vi "ReadVersion.vi"() -> ()   [LabVIEW 2015]
uses:
  <instrlib>/Ion Motion Roboclaw/Ion Motion Roboclaw.lvlib
panel:
  in  "Address":u8
  out "read buffer":string
  out "valid":bool
  in  "baud rate (38400)":u32
  in  "error in (no error)":errorcluster
  out "error out":errorcluster
  in  "COMPort":refnum<visa-resource-name>
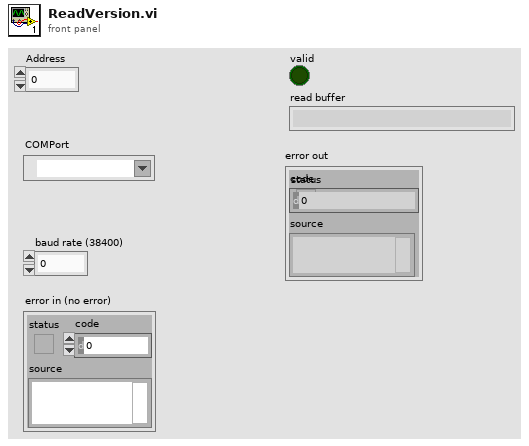
[diagram p1: front panel]
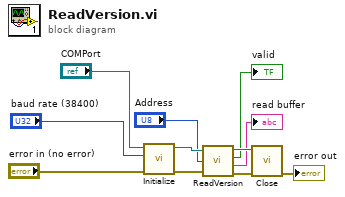
[diagram p0: block diagram]
diagram:
  n1 = call <instrlib>:"Initialize.vi"("error in (no error)"="error in (no error)", "baud rate (38400)"="baud rate (38400)", "COM port"="COMPort") -> ("error out"=w6:errorcluster, "VISA resource name out"=w7:refnum<visa-resource-name>)  [unwired: 7 in]
  n2 = call <instrlib>:"ReadVersion.vi"("VISA Refnum in"=w7, "Address"="Address", "error in (no error)"=w6) -> ("VISA Refnum out"=w5:refnum<visa-resource-name>, "valid"=→"valid":bool, "read buffer"=→"read buffer":string, "error out"=w4:errorcluster)  [unwired: 2 in]
  n3 = call <instrlib>:"Close.vi"("error in (no error)"=w4, "VISA resource name"=w5) -> ("error out"=→"error out":errorcluster)  [unwired: 9 in]
